vi "Is Active.vi"(10 "cycle count":u64=1, 11 "Transfer Group in":refnum<class "Transfer Group.lvclass">) -> (2 "active this cycle?":bool, 3 "Transfer Group out":refnum<class "Transfer Group.lvclass">)   [LabVIEW 2017, in "Data Sharing Framework Core.lvlib" / "Data Sharing Framework Engine.lvlib" / "Transfer Group.lvclass"]
uses:
  Transfer Group.lvclass
  Transfer Group.lvclass/Transfer Group.ctl
  Internal/Timing/Engine Timing.lvclass/Engine Timing.ctl
  Internal/Timing/Get Decimation.vi
  Internal/Timing/Get Offset.vi
  Internal/Timing/Engine Timing.lvclass
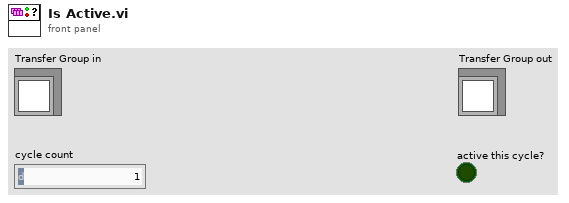
[diagram p1: front panel]
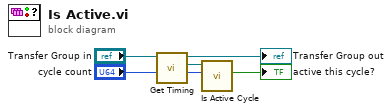
[diagram p0: block diagram]
diagram:
  n1 = call "Get Timing.vi"("Transfer Group in"="Transfer Group in") -> ("Timing"=w4:refnum<class "Engine Timing.lvclass">, "Transfer Group out"=→"Transfer Group out":refnum<class "Transfer Group.lvclass">)  [unwired: 9 in]
  n2 = call "Is Active Cycle.vi"("iteration"="cycle count", "Timing in"=w4) -> ("active?"=→"active this cycle?":bool)  [unwired: 8 in, 1 out]
